vi "Recall Settings From XML File.vi"(2 "error in (no error)":errorcluster, 3 "Controls References":T1, 4 "Settings File Name":string, 5 "Settings File Path":path) -> (0 "error out":errorcluster)   [LabVIEW 2020]
uses:
  Typedefs/Save Settings Control References Control.ctl
  Typedefs/Save settings cluster.ctl
  <vilib>/Utility/xml.llb/Read From XML File(array).vi
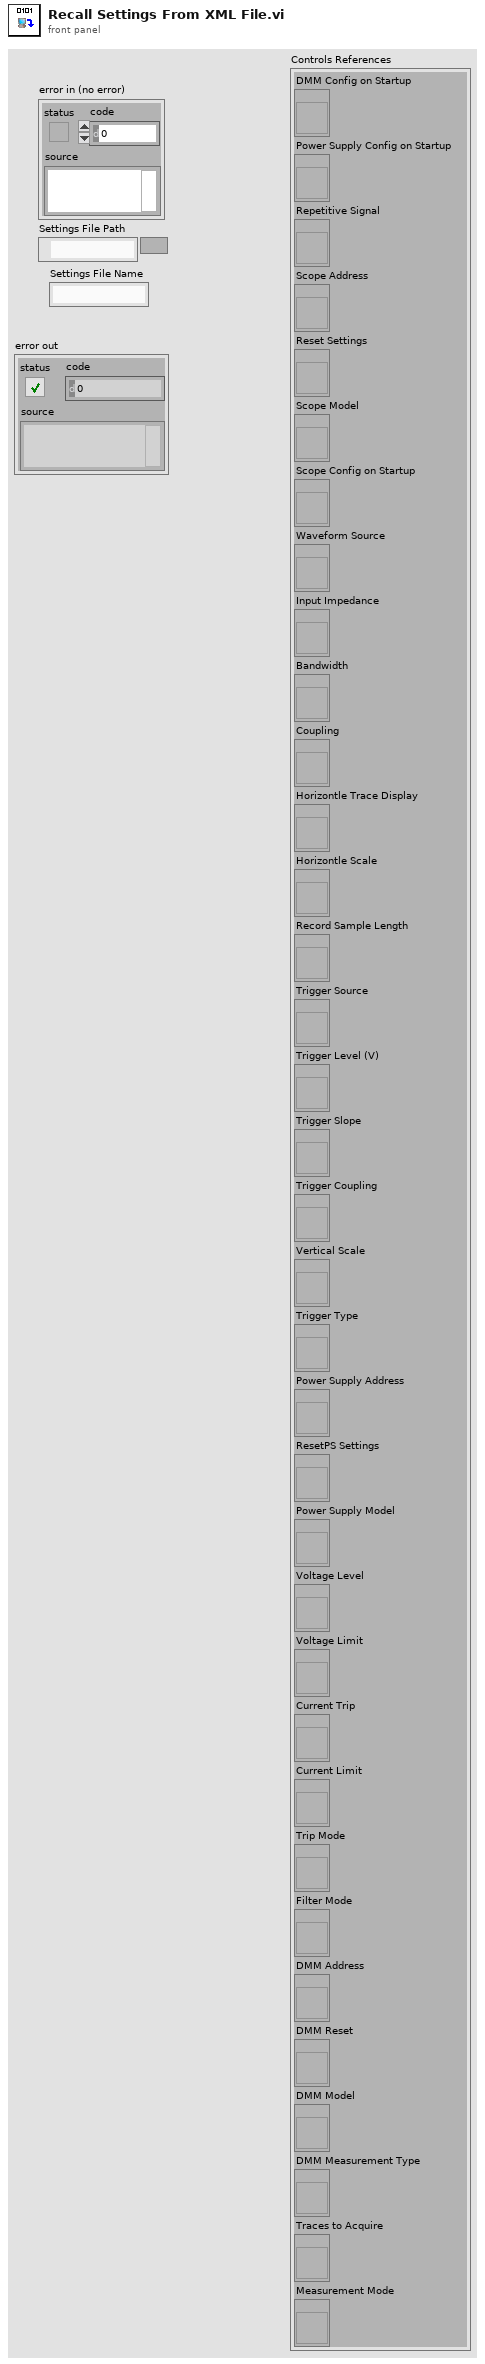
[diagram p1: front panel]
types:
  T1 = typedef "Save Settings Control References Control.ctl" = cluster{"DMM Config on Startup":refnum<vi>, "Power Supply Config on Startup":refnum<vi>, "Repetitive Signal":refnum<vi>, "Scope Address":refnum<vi>, "Reset Settings":refnum<vi>, "Scope Model":refnum<vi>, "Scope Config on Startup":refnum<vi>, "Waveform Source":refnum<vi>, "Input Impedance":refnum<vi>, "Bandwidth":refnum<vi>, "Coupling":refnum<vi>, "Horizontle Trace Display":refnum<vi>, "Horizontle Scale":refnum<vi>, "Record Sample Length":refnum<vi>, "Trigger Source":refnum<vi>, "Trigger Level (V)":refnum<vi>, "Trigger Slope":refnum<vi>, "Trigger Coupling":refnum<vi>, "Vertical Scale":refnum<vi>, "Trigger Type":refnum<vi>, "Power Supply Address":refnum<vi>, "ResetPS Settings":refnum<vi>, "Power Supply Model":refnum<vi>, "Voltage Level":refnum<vi>, "Voltage Limit":refnum<vi>, "Current Trip":refnum<vi>, "Current Limit":refnum<vi>, "Trip Mode":refnum<vi>, "Filter Mode":refnum<vi>, "DMM Address":refnum<vi>, "DMM Reset":refnum<vi>, "DMM Model":refnum<vi>, "DMM Measurement Type":refnum<vi>, "Traces to Acquire":refnum<vi>, "Measurement Mode":refnum<vi>}
  T2 = typedef "Save settings cluster.ctl" = cluster{"Bandwidth":u16, "Coupling":u16, "Current Limit":dbl, "Current Trip":dbl, "DMM Address":refnum<visa-resource-name>, "DMM Measurement Type":i32, "DMM Model":u16, "DMM Reset":bool, "Filter Mode":u16, "Horizontle Scale":i32, "Horizontle Trace Display":i32, "Input Impedance":u16, "Power Supply Address":refnum<visa-resource-name>, "Power Supply Model":enum16{"Keithley 248", "Keithley 237", "Keithley 24XX"}, "Record Sample Length":i32, "Reset Settings":bool, "ResetPS Settings":bool, "Scope Address":refnum<visa-resource-name>, "Scope Config on Startup":u16, "Traces to Acquire":u64, "Trigger Coupling":i32, "Trigger Level (V)":dbl, "Trigger Slope":i32, "Trigger Source":u16, "Trigger Type":u16, "Trip Mode":u16, "Vertical Scale":u16, "Voltage Level":sgl, "Voltage Limit":dbl, "Waveform Source":u16, "Scope Model":u16, "DMM Config on Startup":enum16{"PC->DMM", "DMM->PC"}, "Power Supply Config on Startup":enum16{"PC->Power Supply", "Power Supply->PC"}, "Repetitive Signal":bool, "Measurement Mode":enum16{"Store All Traces in Single File", "Store Average/Std. Dev. for each Point", "Store All Traces in Separate Files"}}
  T3 = enum16{"Store All Traces in Single File", "Store Average/Std. Dev. for each Point", "Store All Traces in Separate Files"}
  T4 = enum16{"Keithley 248", "Keithley 237", "Keithley 24XX"}
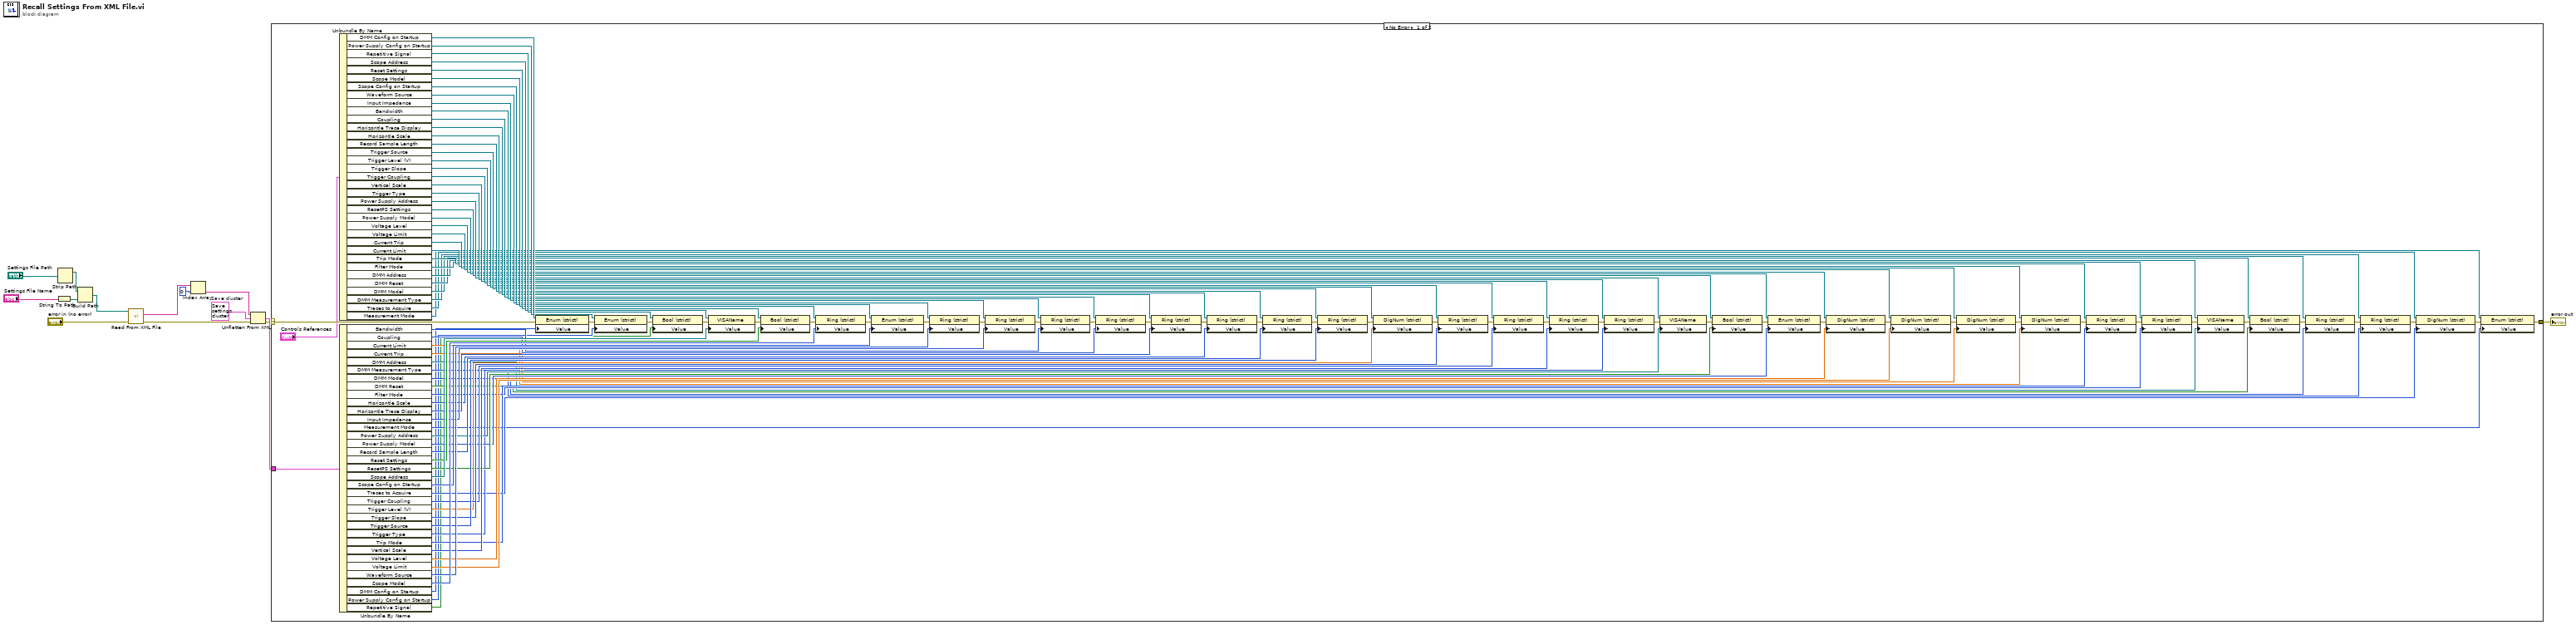
[diagram p0: block diagram]
diagram:
  w10 = T2 {"Bandwidth"=0, "Coupling"=0, "Current Limit"=0.0, "Current Trip"=0.0, "DMM Address"="", "DMM Measurement Type"=0, "DMM Model"=0, "DMM Reset"=FALSE, "Filter Mode"=0, "Horizontle Scale"=0, "Horizontle Trace Display"=0, "Input Impedance"=0, "Power Supply Address"="", "Power Supply Model"=enum."Keithley 248", "Record Sample Length"=0, "Reset Settings"=FALSE, "ResetPS Settings"=FALSE, "Scope Address"="", "Scope Config on Startup"=0, "Traces to Acquire"=0, "Trigger Coupling"=0, "Trigger Level (V)"=0.0, "Trigger Slope"=0, "Trigger Source"=0, "Trigger Type"=0, "Trip Mode"=0, "Vertical Scale"=0, "Voltage Level"=0.0, "Voltage Limit"=0.0, "Waveform Source"=0, "Scope Model"=1, "DMM Config on Startup"=enum."DMM->PC", "Power Supply Config on Startup"=enum."Power Supply->PC", "Repetitive Signal"=FALSE, "Measurement Mode"=enum."Store All Traces in Single File"}  # Save cluster
  n1 = String To Path(string="Settings File Name") -> (path=w4:path)
  n2 = Strip Path(path="Settings File Path") -> (stripped path=w7:path)  [unwired: 1 out]
  n3 = Build Path(base path=w7, name or relative path=w4) -> (appended path=w6:path)
  n4 = call-poly <vilib>:"Read From XML File.vi"("error in (no error)"="error in (no error)", "XML File Path"=w6) -> ("error out"=w12:errorcluster, "XML Elements"=w13:string[])  [unwired: 7 in, 1 out]
  n5 = Index Array(array=w13, index=0) -> (element=w11:string)
  n6 = Unflatten From XML(xml string=w11, type=w10, error in (no error)=w12) -> (value=w9:T2, error out=w8:errorcluster)
  n7 = case shown="No Error" w8 {
    selector: w8 -> [w54 w123]
    tunnel: w9 -> [w122 _]
    tunnel: [w58 w123] -> w1
    frame No Error {
      n8 = Unbundle By Name("Controls References") -> ("DMM Config on Startup"=w49:refnum<vi>, "Power Supply Config on Startup"=w48:refnum<vi>, "Repetitive Signal"=w47:refnum<vi>, "Scope Address"=w46:refnum<vi>, "Reset Settings"=w45:refnum<vi>, "Scope Model"=w44:refnum<vi>, "Scope Config on Startup"=w43:refnum<vi>, "Waveform Source"=w42:refnum<vi>, "Input Impedance"=w41:refnum<vi>, "Bandwidth"=w40:refnum<vi>, "Coupling"=w39:refnum<vi>, "Horizontle Trace Display"=w38:refnum<vi>, "Horizontle Scale"=w37:refnum<vi>, "Record Sample Length"=w36:refnum<vi>, "Trigger Source"=w35:refnum<vi>, "Trigger Level (V)"=w34:refnum<vi>, "Trigger Slope"=w33:refnum<vi>, "Trigger Coupling"=w32:refnum<vi>, "Vertical Scale"=w31:refnum<vi>, "Trigger Type"=w30:refnum<vi>, "Power Supply Address"=w29:refnum<vi>, "ResetPS Settings"=w28:refnum<vi>, "Power Supply Model"=w27:refnum<vi>, "Voltage Level"=w26:refnum<vi>, "Voltage Limit"=w25:refnum<vi>, "Current Trip"=w24:refnum<vi>, "Current Limit"=w23:refnum<vi>, "Trip Mode"=w22:refnum<vi>, "Filter Mode"=w21:refnum<vi>, "DMM Address"=w20:refnum<vi>, "DMM Reset"=w19:refnum<vi>, "DMM Model"=w18:refnum<vi>, "DMM Measurement Type"=w17:refnum<vi>, "Traces to Acquire"=w16:refnum<vi>, "Measurement Mode"=w15:refnum<vi>)
      n9 = Unbundle By Name(w122) -> ("Bandwidth"=w101:u16, "Coupling"=w100:u16, "Current Limit"=w76:dbl, "Current Trip"=w77:dbl, "DMM Address"=w64:refnum<visa-resource-name>, "DMM Measurement Type"=w61:i32, "DMM Model"=w62:u16, "DMM Reset"=w63:bool, "Filter Mode"=w71:u16, "Horizontle Scale"=w98:i32, "Horizontle Trace Display"=w99:i32, "Input Impedance"=w102:u16, "Measurement Mode"=w59:T3, "Power Supply Address"=w88:refnum<visa-resource-name>, "Power Supply Model"=w86:T4, "Record Sample Length"=w97:i32, "Reset Settings"=w119:bool, "ResetPS Settings"=w87:bool, "Scope Address"=w121:refnum<visa-resource-name>, "Scope Config on Startup"=w115:u16, "Traces to Acquire"=w60:u64, "Trigger Coupling"=w94:i32, "Trigger Level (V)"=w93:dbl, "Trigger Slope"=w95:i32, "Trigger Source"=w96:u16, "Trigger Type"=w72:u16, "Trip Mode"=w75:u16, "Vertical Scale"=w92:u16, "Voltage Level"=w79:sgl, "Voltage Limit"=w78:dbl, "Waveform Source"=w103:u16, "Scope Model"=w118:u16, "DMM Config on Startup"=w57:enum16{"PC->DMM", "DMM->PC"}, "Power Supply Config on Startup"=w55:enum16{"PC->Power Supply", "Power Supply->PC"}, "Repetitive Signal"=w52:bool)
      n10 = property on="Property Node" class="Enum (strict)"(reference=w49, error in=w54, "Value"=w57) -> (error out=w56:errorcluster)  [unwired: 1 out]
      n11 = property on="Property Node" class="Enum (strict)"(reference=w48, error in=w56, "Value"=w55) -> (error out=w53:errorcluster)  [unwired: 1 out]
      n12 = property on="Property Node" class="Bool (strict)"(reference=w47, error in=w53, "Value"=w52) -> (error out=w51:errorcluster)  [unwired: 1 out]
      n13 = property on="Property Node" class="VISAName"(reference=w46, error in=w51, "Value"=w121) -> (error out=w120:errorcluster)  [unwired: 1 out]
      n14 = property on="Property Node" class="Bool (strict)"(reference=w45, error in=w120, "Value"=w119) -> (error out=w117:errorcluster)  [unwired: 1 out]
      n15 = property on="Property Node" class="Ring (strict)"(reference=w44, error in=w117, "Value"=w118) -> (error out=w116:errorcluster)  [unwired: 1 out]
      n16 = property on="Property Node" class="Enum (strict)"(reference=w43, error in=w116, "Value"=w115) -> (error out=w111:errorcluster)  [unwired: 1 out]
      n17 = property on="Property Node" class="Ring (strict)"(reference=w42, error in=w111, "Value"=w103) -> (error out=w112:errorcluster)  [unwired: 1 out]
      n18 = property on="Property Node" class="Ring (strict)"(reference=w41, error in=w112, "Value"=w102) -> (error out=w110:errorcluster)  [unwired: 1 out]
      n19 = property on="Property Node" class="Ring (strict)"(reference=w40, error in=w110, "Value"=w101) -> (error out=w109:errorcluster)  [unwired: 1 out]
      n20 = property on="Property Node" class="Ring (strict)"(reference=w39, error in=w109, "Value"=w100) -> (error out=w108:errorcluster)  [unwired: 1 out]
      n21 = property on="Property Node" class="Ring (strict)"(reference=w38, error in=w108, "Value"=w99) -> (error out=w113:errorcluster)  [unwired: 1 out]
      n22 = property on="Property Node" class="Ring (strict)"(reference=w37, error in=w113, "Value"=w98) -> (error out=w114:errorcluster)  [unwired: 1 out]
      n23 = property on="Property Node" class="Ring (strict)"(reference=w36, error in=w114, "Value"=w97) -> (error out=w91:errorcluster)  [unwired: 1 out]
      n24 = property on="Property Node" class="Ring (strict)"(reference=w35, error in=w91, "Value"=w96) -> (error out=w107:errorcluster)  [unwired: 1 out]
      n25 = property on="Property Node" class="DigNum (strict)"(reference=w34, error in=w107, "Value"=w93) -> (error out=w106:errorcluster)  [unwired: 1 out]
      n26 = property on="Property Node" class="Ring (strict)"(reference=w33, error in=w106, "Value"=w95) -> (error out=w105:errorcluster)  [unwired: 1 out]
      n27 = property on="Property Node" class="Ring (strict)"(reference=w32, error in=w105, "Value"=w94) -> (error out=w104:errorcluster)  [unwired: 1 out]
      n28 = property on="Property Node" class="Ring (strict)"(reference=w31, error in=w104, "Value"=w92) -> (error out=w74:errorcluster)  [unwired: 1 out]
      n29 = property on="Property Node" class="Ring (strict)"(reference=w30, error in=w74, "Value"=w72) -> (error out=w73:errorcluster)  [unwired: 1 out]
      n30 = property on="Property Node" class="VISAName"(reference=w29, error in=w73, "Value"=w88) -> (error out=w90:errorcluster)  [unwired: 1 out]
      n31 = property on="Property Node" class="Bool (strict)"(reference=w28, error in=w90, "Value"=w87) -> (error out=w89:errorcluster)  [unwired: 1 out]
      n32 = property on="Property Node" class="Enum (strict)"(reference=w27, error in=w89, "Value"=w86) -> (error out=w85:errorcluster)  [unwired: 1 out]
      n33 = property on="Property Node" class="DigNum (strict)"(reference=w26, error in=w85, "Value"=w79) -> (error out=w84:errorcluster)  [unwired: 1 out]
      n34 = property on="Property Node" class="DigNum (strict)"(reference=w25, error in=w84, "Value"=w78) -> (error out=w83:errorcluster)  [unwired: 1 out]
      n35 = property on="Property Node" class="DigNum (strict)"(reference=w24, error in=w83, "Value"=w77) -> (error out=w82:errorcluster)  [unwired: 1 out]
      n36 = property on="Property Node" class="DigNum (strict)"(reference=w23, error in=w82, "Value"=w76) -> (error out=w81:errorcluster)  [unwired: 1 out]
      n37 = property on="Property Node" class="Ring (strict)"(reference=w22, error in=w81, "Value"=w75) -> (error out=w80:errorcluster)  [unwired: 1 out]
      n38 = property on="Property Node" class="Ring (strict)"(reference=w21, error in=w80, "Value"=w71) -> (error out=w70:errorcluster)  [unwired: 1 out]
      n39 = property on="Property Node" class="VISAName"(reference=w20, error in=w70, "Value"=w64) -> (error out=w69:errorcluster)  [unwired: 1 out]
      n40 = property on="Property Node" class="Bool (strict)"(reference=w19, error in=w69, "Value"=w63) -> (error out=w68:errorcluster)  [unwired: 1 out]
      n41 = property on="Property Node" class="Ring (strict)"(reference=w18, error in=w68, "Value"=w62) -> (error out=w67:errorcluster)  [unwired: 1 out]
      n42 = property on="Property Node" class="Ring (strict)"(reference=w17, error in=w67, "Value"=w61) -> (error out=w66:errorcluster)  [unwired: 1 out]
      n43 = property on="Property Node" class="DigNum (strict)"(reference=w16, error in=w66, "Value"=w60) -> (error out=w65:errorcluster)  [unwired: 1 out]
      n44 = property on="Property Node" class="Enum (strict)"(reference=w15, error in=w65, "Value"=w59) -> (error out=w58:errorcluster)  [unwired: 1 out]
    }
    frame Error {
    }
  }
  "error out" <- w1
